vi "UnboxBoolean.vi"(10 "Boolean in":refnum<class "Boolean.lvclass">) -> (2 "Boolean":bool)   [LabVIEW 2013, in "LapDog.Collections.v_.Common.lvlib" / "Boolean.lvclass"]
uses:
  Boolean.lvclass
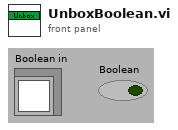
[diagram p1: front panel]
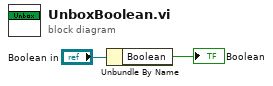
[diagram p0: block diagram]
diagram:
  n1 = Unbundle By Name("Boolean in") -> ("Boolean"=→"Boolean":bool)
